vi "Generate Waveform Path.vi"(1 "Relative Waveform Path":string, 2 "Target Name":string) -> (0 "Waveform Path Out":string)   [LabVIEW 2019, in "FPGA Addon Test Class.lvclass"]
uses:
  FPGA Addon Test Class.lvclass
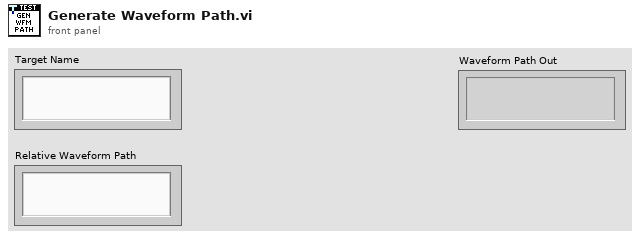
[diagram p1: front panel]
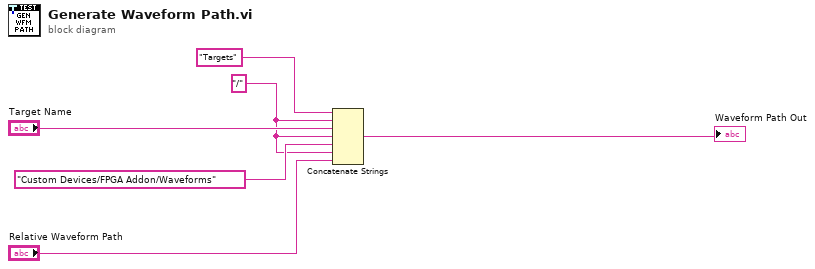
[diagram p0: block diagram]
diagram:
  w3 = "/" ("string")
  n1 = Concatenate Strings("Targets" ("string"), w3, "Target Name", w3, "Custom Devices/FPGA Addon/Waveforms" ("string"), w3, "Relative Waveform Path") -> (→"Waveform Path Out":string)
